vi "test Enum.vi"() -> ()   [LabVIEW 2017]
uses:
  addons/API-String-Arugments-Support/API String Arguments Support.lvlib
panel:
  out "data":enum16{"5", "2", "33"}(ring)
  out "Enum":variant
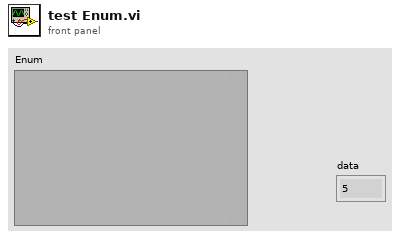
[diagram p1: front panel]
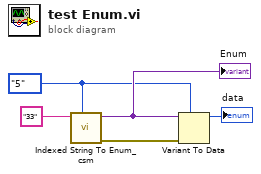
[diagram p0: block diagram]
diagram:
  w2 = enum16{"5", "2", "33"}."5"
  n1 = call "Indexed String To Enum_csm.vi"("Variant"=w2, "String"="33") -> ("error out"=w4:errorcluster, "Enum"=w3:variant)  [unwired: 8 in]
  "Enum" <- w3
  n2 = Variant To Data(error in=w4, type=w2, Variant=w3) -> (data=→"data":enum16{"5", "2", "33"})  [unwired: 1 out]
